vi "Auto width colum table.vi"(9 "error in (no error)":errorcluster, 10 "spazi":i16=27, 11 "Real Time tabella":refnum<vi>) -> (1 "error out":errorcluster)   [LabVIEW 2019]
uses:
  <vilib>/Utility/miscctls.llb/LVRowAndColumnTypeDef.ctl
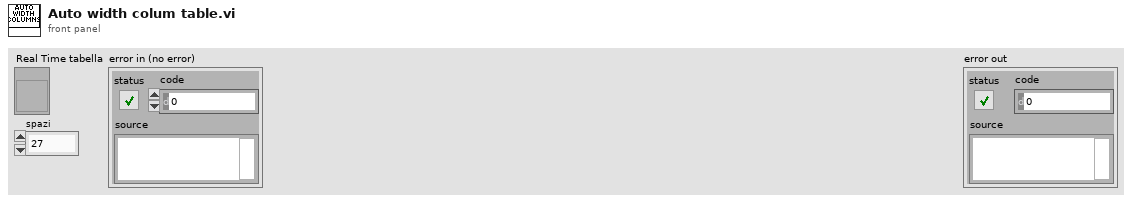
[diagram p1: front panel]
types:
  T1 = cluster{"Font Name:":string, "Size":i16, "Strikeout?":bool, "Italic?":bool, "Underline?":bool, "Outline?":bool, "Shadow?":bool, "Bold?":bool}
  T2 = typedef "LVRowAndColumnTypeDef.ctl" = cluster{"Row":i32, "Column":i32}
  T3 = enum16{"User-specified Font", "Application Font", "System Font", "Dialog Font"}
  T4 = cluster{"left":i16, "top":i16, "right":i16, "bottom":i16}
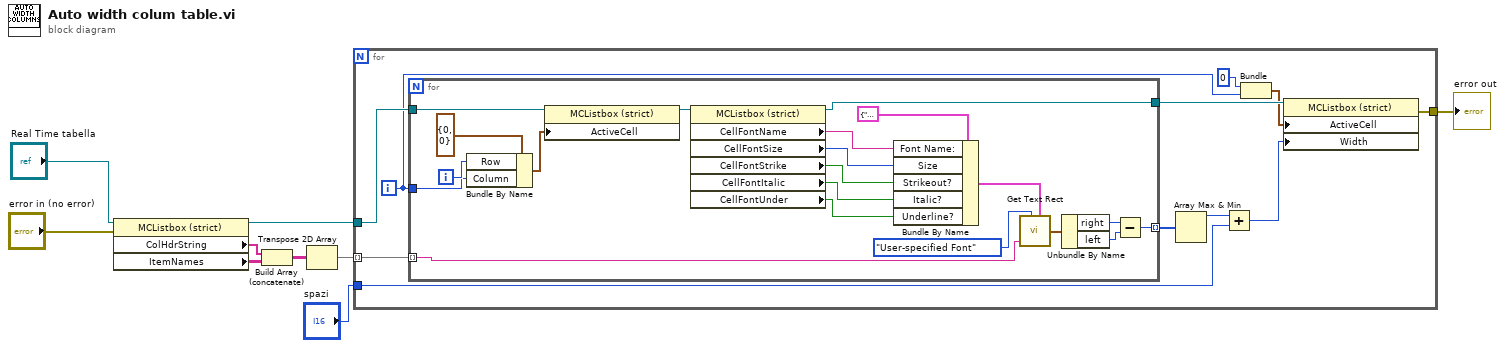
[diagram p0: block diagram]
diagram:
  n1 = property class="MCListbox (strict)"(reference="Real Time tabella", error in="error in (no error)") -> (reference out=w7:refnum<vi>, "ColHdrString"=w3:string[], "ItemNames"=w9:string[][])  [unwired: 1 out]
  n2 = Build Array (concatenate)(w3, w9) -> (w4:string[][])
  n3 = Transpose 2D Array(2D array=w4) -> (transposed array=w8:string[][])
  n4 = for {
    tunnel: w8 -> [w20] mode=indexing
    tunnel: w7 -> [w19]
    tunnel: [w11] -> w2
    tunnel: "spazi" -> [w10]
    i -> [w15]
    n5 = for {
      tunnel: w20 -> [w39] mode=indexing
      tunnel: [w35] -> w18 mode=indexing
      tunnel: w19 -> [w34]
      tunnel: w15 -> [w30]
      tunnel: [w21] -> w16
      i -> [w31]
      n6 = Bundle By Name(cluster=T2 {"Row"=0, "Column"=0} ("Active Cell:Active Cell"), "Row"=w31, "Column"=w30) -> (w32:T2)
      n7 = property class="MCListbox (strict)"(reference=w34, "ActiveCell"=w32) -> (reference out=w28:refnum<vi>)  [unwired: 1 in, 1 out]
      n8 = property class="MCListbox (strict)"(reference=w28) -> (reference out=w21:refnum<vi>, "CellFontName"=w27:string, "CellFontSize"=w26:u32, "CellFontStrike"=w25:bool, "CellFontItalic"=w23:bool, "CellFontUnder"=w22:bool)  [unwired: 1 in, 1 out]
      n9 = Bundle By Name(cluster=T1 {"Font Name:"="sadsad", "Size"=4, "Strikeout?"=FALSE, "Italic?"=FALSE, "Underline?"=FALSE, "Outline?"=FALSE, "Shadow?"=FALSE, "Bold?"=FALSE} ("[user-specified font]"), "Font Name:"=w27, "Size"=w26, "Strikeout?"=w25, "Italic?"=w23, "Underline?"=w22) -> (w24:T1)
      n10 = call <vilib>:"Get Text Rect.vi"("desired font(Application)"=T3."User-specified Font", "text"=w39, "[user-specified font]"=w24) -> ("rect"=w38:T4)  [unwired: 6 in]
      n11 = Unbundle By Name(w38) -> ("right"=w36:i16, "left"=w37:i16)
      n12 = Subtract(x=w36, y=w37) -> (x-y=w35:i16)
    }
    n13 = Array Max & Min(array=w18) -> (max value=w17:i16)  [unwired: 3 out]
    n14 = Add(x=w17, y=w10) -> (x+y=w12:i16)
    n15 = Bundle("y"=i16 0, w15) -> (w13:cluster{"y":i16, i32})  [unwired: 1 in]
    n16 = property class="MCListbox (strict)"(reference=w16, "ActiveCell"=w13, "Width"=w12) -> (error out=w11:errorcluster)  [unwired: 1 in, 1 out]
  }
  "error out" <- w2
